vi "Reset Auton.vi"() -> (3 "Reset Auton":bool)   [LabVIEW 2014]
uses:
  <vilib>/Rock Robotics/WPI/DriverStation/WPI_DriverStationRobotMode2.ctl
  <vilib>/Rock Robotics/Network Tables/SD Read Boolean.vi
  Begin/Global Variables.vi
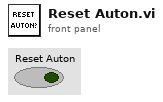
[diagram p1: front panel]
types:
  T1 = typedef "WPI_DriverStationRobotMode2.ctl" = enum16{"Autonomous Disabled", "Autonomous Enabled", "Teleop Disabled", "Teleop Enabled", "Disconnected", "Finish", "Test Disabled", "Test Enabled", "Emergency Stopped"}
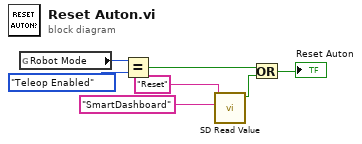
[diagram p0: block diagram]
diagram:
  n1 = global read "Global Variables.vi" "Robot Mode"() -> (w4:T1)
  n2 = Equal?(x=w4, y=WPI_DriverStationRobotMode2."Teleop Enabled") -> (x = y?=w3:bool)
  n3 = call-poly <vilib>:"SD Read Value.vi"("Table Prefix"="SmartDashboard", "Name"="Reset") -> ("Boolean"=w2:bool)  [unwired: 7 in, 2 out]
  n4 = Or(x=w3, y=w2) -> (x .or. y?=→"Reset Auton":bool)
